vi "mWmotor_set_Count.vi"(8 "error in (no error)":errorcluster, 10 "Revolutions":dbl, 11 "VISA resource name":refnum<visa-resource-name>) -> (0 "error out":errorcluster, 3 "VISA resource name out":refnum<visa-resource-name>)   [LabVIEW 2019]
panel:
  in  "milliseconds to wait":u32=100
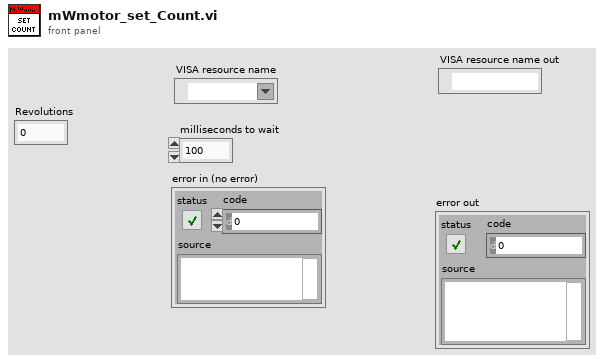
[diagram p1: front panel]
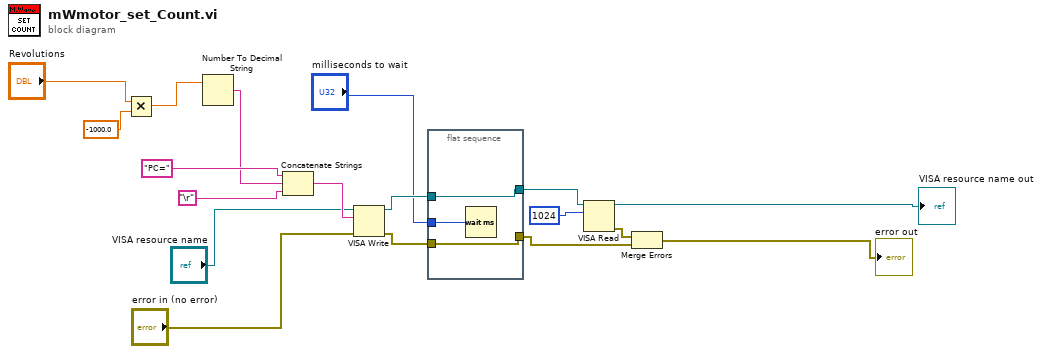
[diagram p0: block diagram]
diagram:
  n1 = Multiply(x="Revolutions", y=-1000.0) -> (x*y=w3:dbl)
  n2 = Number To Decimal String(number=w3) -> (decimal integer string=w1:string)  [unwired: 1 in]
  n3 = Concatenate Strings("PC=" ("string"), w1, "\r") -> (w18:string)
  n4 = VISA Write(VISA resource name="VISA resource name", write buffer=w18, error in (no error)="error in (no error)") -> (VISA resource name out=w14:refnum<visa-resource-name>, error out=w15:errorcluster)  [unwired: 1 out]
  n5 = flat-sequence {
    tunnel: [w21] -> w10
    tunnel: w15 -> [w21]
    tunnel: [w20] -> w13
    tunnel: w14 -> [w20]
    tunnel: "milliseconds to wait" -> [w19]
    frame #0 {
      n6 = Wait (ms)(milliseconds to wait=w19) -> ()  [unwired: 1 out]
    }
  }
  n7 = VISA Read(VISA resource name=w13, byte count=u32 1024) -> (VISA resource name out=→"VISA resource name out":refnum<visa-resource-name>, error out=w9:errorcluster)  [unwired: 1 in, 2 out]
  n8 = Merge Errors(w9, w10) -> (→"error out":errorcluster)
